vi "YAV分贝计算.vi"(11 "子数组输入":dbl[](array[numeric])) -> (3 "f":dbl)   [LabVIEW 2011]
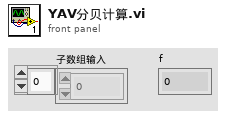
[diagram p1: front panel]
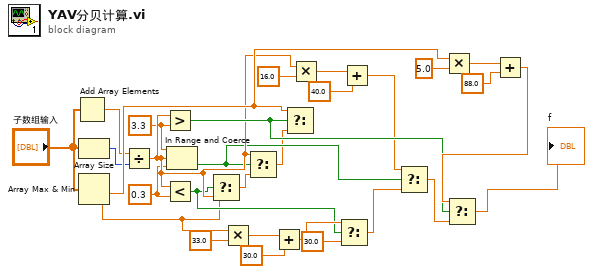
[diagram p0: block diagram]
diagram:
  w6 = 3.3 ("上限")
  w4 = 0.3 ("y")
  n1 = Add Array Elements(numeric array="子数组输入") -> (sum=w1:dbl)
  n2 = Array Size(array="子数组输入") -> (size(s)=w2:i32)
  n3 = Array Max & Min(array="子数组输入") -> (max value=w8:dbl, min value=w25:dbl)  [unwired: 2 out]
  n4 = Divide(x=w1, y=w2) -> (x/y=w21:dbl)
  n5 = Greater?(x=w21, y=w6) -> (0:w26:bool)
  n6 = Less?(x=w21, y=w4) -> (x < y?=w12:bool)
  n7 = In Range and Coerce(upper limit=w6, x=w21, lower limit=w4) -> (In Range?=w15:bool)  [unwired: 1 out]
  n8 = Select(t=w8, s=w12, f=w21) -> (s? t:f=w5:dbl)
  n9 = Multiply(x=w8, y=33.0) -> (x*y=w10:dbl)
  n10 = Select(t=w21, s=w15, f=w5) -> (s? t:f=w7:dbl)
  n11 = Add(x=w10, y=30.0) -> (x+y=w13:dbl)
  n12 = Select(t=w25, s=w26, f=w7) -> ()  [unwired: 1 out]
  n13 = Multiply(x=w21, y=16.0) -> (x*y=w18:dbl)
  n14 = Select(t=w13, s=w12, f=30.0) -> (s? t:f=w16:dbl)
  n15 = Add(x=w18, y=40.0) -> (x+y=w20:dbl)
  n16 = Select(t=w20, s=w15, f=w16) -> (s? t:f=w28:dbl)
  n17 = Multiply(x=w25, y=5.0) -> (x*y=w23:dbl)
  n18 = Add(x=w23, y=88.0) -> (x+y=w27:dbl)
  n19 = Select(t=w27, s=w26, f=w28) -> (s? t:f=→"f":dbl)
